vi "DataFrontPanelRead.vi"(0 "SR865 in":T2, 2 "DataFrontPanel":T1=2 caption="Data channel" items=["Green", "Blue", "Yellow", "Orange"], 5 "error in":errorcluster) -> (14 "SR865 out":T2, 16 "Data":dbl, 19 "error out":errorcluster)   [LabVIEW 2017]
uses:
  SR865.ctl
  DataFrontPanel.ctl
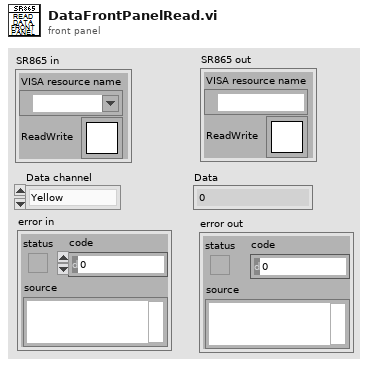
[diagram p1: front panel]
types:
  T1 = typedef "DataFrontPanel.ctl" = u16
  T2 = typedef "SR865.ctl" = cluster{"VISA resource name":refnum<visa-resource-name>, "ReadWrite":T3}
  T3 = typedef "Semaphore RefNum" = refnum<k1>
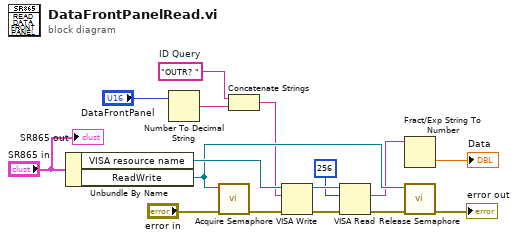
[diagram p0: block diagram]
diagram:
  w4 = "OUTR? "  # ID Query
  n1 = Unbundle By Name("SR865 in") -> ("VISA resource name"=w12:refnum<visa-resource-name>, "ReadWrite"=w7:T3)
  n2 = Number To Decimal String(number="DataFrontPanel") -> (decimal integer string=w1:string)  [unwired: 1 in]
  n3 = call <vilib>:"Acquire Semaphore.vi"("error in (no error)"="error in", "semaphore"=w7) -> ("error out"=w11:errorcluster)  [unwired: 3 in, 2 out]
  n4 = Concatenate Strings(w4, w1) -> (w3:string)
  n5 = VISA Write(VISA resource name=w12, write buffer=w3, error in (no error)=w11) -> (VISA resource name out=w15:refnum<visa-resource-name>, error out=w14:errorcluster)  [unwired: 1 out]
  n6 = VISA Read(VISA resource name=w15, byte count=u32 256, error in (no error)=w14) -> (read buffer=w6:string, error out=w9:errorcluster)  [unwired: 2 out]
  n7 = Fract/Exp String To Number(string=w6) -> (number=→"Data":dbl)  [unwired: 3 in, 1 out]
  n8 = call <vilib>:"Release Semaphore.vi"("error in (no error)"=w9, "semaphore"=w7) -> ("error out"=→"error out":errorcluster)  [unwired: 4 in, 1 out]
  "SR865 out" <- "SR865 in"
